vi "Init Target Instrument.vi"(8 "error in":errorcluster, 9 "<JSON CFG>":string, 10 "Physical Instr CFGs":string[](array[string]), 11 "Target MSS in":refnum<class "CRIO MSS Test Actor.lvclass">) -> (0 "error out":errorcluster, 3 "Target MSS out":refnum<class "CRIO MSS Test Actor.lvclass">)   [LabVIEW 2023, in "CRIO MSS Test Actor.lvlib" / "CRIO MSS Test Actor.lvclass"]
uses:
  CRIO MSS Test Actor.lvclass
  CRIO MSS Test Actor.lvclass/CRIO MSS Test Actor.ctl
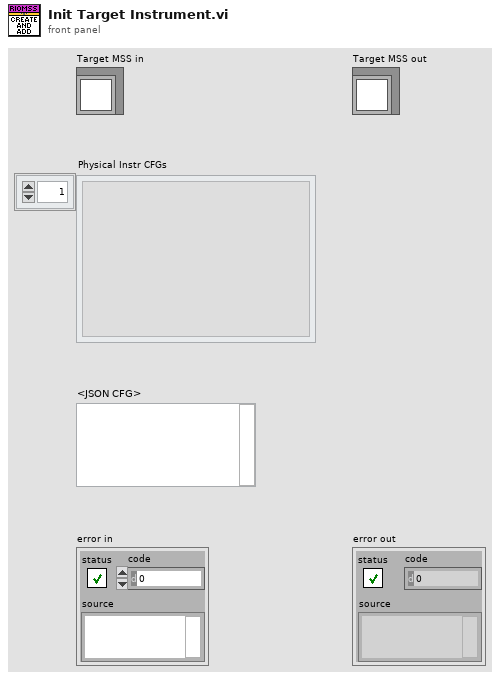
[diagram p1: front panel]
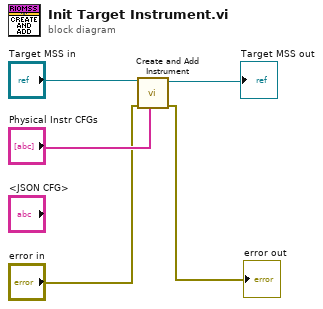
[diagram p0: block diagram]
diagram:
  n1 = call-dynamic "Create and Add Instrument.vi"("Physical Instr CFGs"="Physical Instr CFGs", "error in"="error in", "Target MSS in"="Target MSS in") -> ("error out"=→"error out":errorcluster, "Target MSS out"=→"Target MSS out":refnum<class "CRIO MSS Test Actor.lvclass">)  [unwired: 7 in]
